vi "Data Queue2.vi"(5 "timeout in ms (-1)":i32=10, 6 "max queue size (-1, unlimited)":i32, 7 "Action":T1=enum."Enqueue", 8 "error in (no error)":errorcluster, 11 "data in":sgl[](array[numeric])) -> (0 "error out":errorcluster, 1 "Empty?":bool, 2 "# elements in queue":i32, 3 "data out":sgl[](array[numeric]))   [LabVIEW 2018]
uses:
  Controls/Queue Manager Actions.ctl
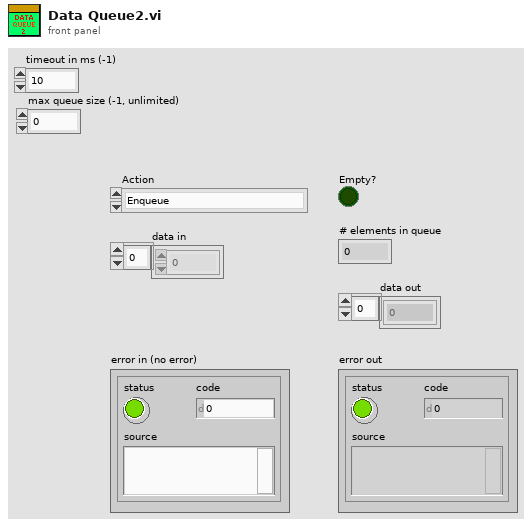
[diagram p1: front panel]
types:
  T1 = typedef "Queue Manager Actions.ctl" = enum16{"Init", "Enqueue", "Enqueue All", "Preview Queue", "Dequeue", "Get Status", "Flush Queue", "Flush All Queues", "Release All Queues", "Release Queue", "Enqueue at Opposite End"}
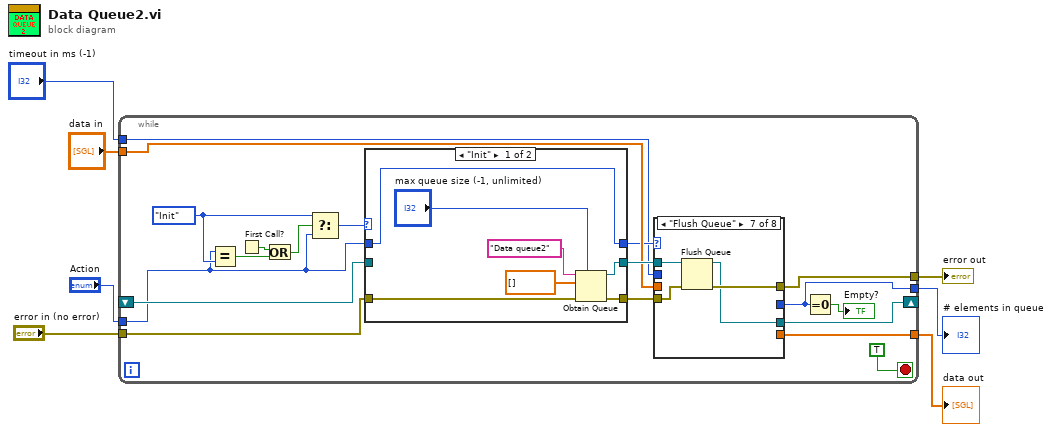
[diagram p0: block diagram]
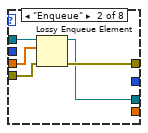
[diagram p3: hidden frame]
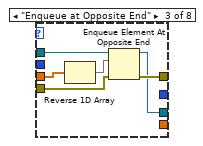
[diagram p4: hidden frame]
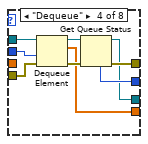
[diagram p5: hidden frame]
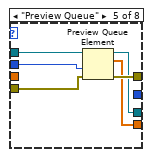
[diagram p6: hidden frame]
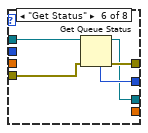
[diagram p7: hidden frame]
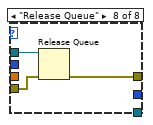
[diagram p8: hidden frame]
diagram:
  n1 = while {
    tunnel: "Action" -> [w9]
    tunnel: "error in (no error)" -> [w14]
    shift-right: [w16] -> _
    shift-left: _ -> [w15]
    tunnel: "data in" -> [w12]
    tunnel: "timeout in ms (-1)" -> [w8]
    tunnel: [w19] -> w3
    tunnel: [w18] -> w2
    tunnel: [w11] -> w1
    stop <- TRUE stop-if-true
    w21 = Queue_Manager_Actions."Init"
    n2 = Equal?(x=w9, y=w21) -> (x = y?=w23:bool)
    n3 = First Call?() -> (First Call?: T/F=w24:bool)
    n4 = Or(x=w24, y=w23) -> (x .or. y?=w22:bool)
    n5 = Select(t=w21, s=w22, f=w9) -> (s? t:f=w20:T1)
    n6 = case shown="\"Init\"" w20 {
      tunnel: [w73 w76] -> w17
      tunnel: [w72 w75] -> w13
      tunnel: w15 -> [_ w76]
      tunnel: w14 -> [w70 w75]
      tunnel: [w68 w74] -> w10
      tunnel: w9 -> [w68 w74]
      frame "Init" {
        n7 = Obtain Queue(max queue size (-1, unlimited)="max queue size (-1, unlimited)", name (unnamed)="Data queue2", element data type=sgl[] [], error in (no error)=w70) -> (queue out=w73:refnum<queue>, error out=w72:errorcluster)  [unwired: 1 in, 1 out]
      }
      frame Default {
      }
    }
    n8 = case shown="\"Flush Queue\"" w10 {
      tunnel: [w27 w33 w39 w47 w54 w59 w63 w66] -> w19
      tunnel: [_ _ _ w44 w53 _ _ _] -> w18
      tunnel: [_ _ _ w45 _ w58 _ _] -> w11
      tunnel: w17 -> [w28 w32 w36 w43 w51 w57 w62 w65]
      tunnel: [w28 w29 w37 w41 w50 w55 w60 _] -> w16
      tunnel: w13 -> [w27 w31 w35 w42 w52 w56 w61 w64]
      tunnel: w12 -> [_ w30 w34 _ _ _ _ _]
      tunnel: w8 -> [_ _ _ w40 w49 _ _ _]
      frame "Init", Default {
      }
      frame "Enqueue" {
        n9 = Lossy Enqueue Element(queue=w32, element=w30, error in (no error)=w31) -> (queue out=w29:refnum<queue>, error out=w33:errorcluster)  [unwired: 2 out]
      }
      frame "Enqueue at Opposite End" {
        n10 = Reverse 1D Array(array=w34) -> (reversed array=w38:sgl[])
        n11 = Enqueue Element At Opposite End(queue=w36, element=w38, error in (no error)=w35) -> (queue out=w37:refnum<queue>, error out=w39:errorcluster)  [unwired: 1 in, 1 out]
      }
      frame "Dequeue" {
        n12 = Dequeue Element(queue=w43, timeout in ms (-1)=w40, error in (no error)=w42) -> (queue out=w46:refnum<queue>, element=w44:sgl[], error out=w48:errorcluster)  [unwired: 1 out]
        n13 = Get Queue Status(queue=w46, error in (no error)=w48) -> (queue out=w41:refnum<queue>, error out=w47:errorcluster, # elements in queue=w45:i32)  [unwired: 1 in, 5 out]
      }
      frame "Preview Queue" {
        n14 = Preview Queue Element(queue=w51, timeout in ms (-1)=w49, error in (no error)=w52) -> (queue out=w50:refnum<queue>, element=w53:sgl[], error out=w54:errorcluster)  [unwired: 1 out]
      }
      frame "Get Status" {
        n15 = Get Queue Status(queue=w57, error in (no error)=w56) -> (queue out=w55:refnum<queue>, error out=w59:errorcluster, # elements in queue=w58:i32)  [unwired: 1 in, 5 out]
      }
      frame "Flush Queue" {
        n16 = Flush Queue(queue=w62, error in (no error)=w61) -> (queue out=w60:refnum<queue>, error out=w63:errorcluster)  [unwired: 1 out]
      }
      frame "Release Queue" {
        n17 = Release Queue(queue=w65, error in (no error)=w64) -> (error out=w66:errorcluster)  [unwired: 1 in, 2 out]
      }
    }
    n18 = Equal To 0?(x=w11) -> (x = 0?=→"Empty?":bool)
  }
  "error out" <- w3
  "data out" <- w2
  "# elements in queue" <- w1
